vi "WFS Error Message.vi"(8 "error in (no error)":errorcluster {"code" format="%.0x"}, 10 "Error Code":i32 format="%.0g", 11 "instrument handle":refnum<visa-resource-name>) -> (0 "error out":errorcluster {"code" format="%.0x"}, 2 "Error Message":string, 3 "instrument handle out":refnum<visa-resource-name>)   [LabVIEW 2020]
doc: "This VI translates the error return value from a VXIplug&play instrument driver VI to a user-readable string."
uses:
  WFS_32.dll
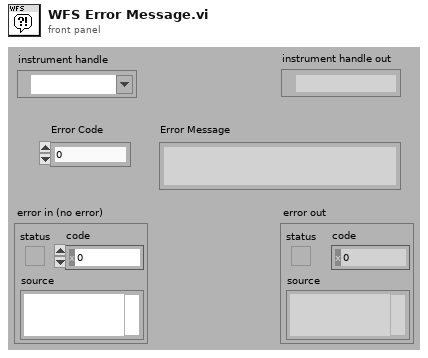
[diagram p1: front panel]
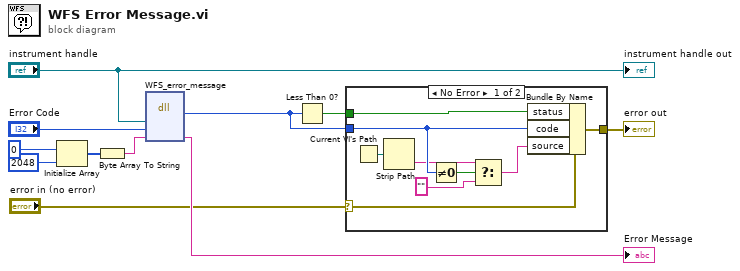
[diagram p0: block diagram]
diagram:
  n1 = Initialize Array(u8 0, 2048 ("size of error message")) -> (w9:u8[])
  n2 = Byte Array To String(unsigned byte array=w9) -> (string=w7:string)
  n3 = dll-call lib="WFS_*.*" fn="WFS_error_message"("instrument handle"="instrument handle", "error code"="Error Code", "error message"=w7) -> ("Status"=w2:i32, "error message"=→"Error Message":string)  [unwired: 5 in, 2 out]
  n4 = Less Than 0?(x=w2) -> (x < 0?=w3:bool)
  n5 = case shown="No Error" "error in (no error)" {
    selector: "error in (no error)" -> [w15 w21]
    tunnel: [w17 w21] -> w1
    tunnel: w3 -> [w18 _]
    tunnel: w2 -> [w14 _]
    frame No Error {
      n6 = Current VI's Path() -> (path=w13:path)
      n7 = Strip Path(path=w13) -> (name=w12:string)  [unwired: 1 out]
      n8 = Not Equal To 0?(x=w14) -> (x != 0?=w16:bool)
      n9 = Select(t=w12, s=w16, f="") -> (s? t:f=w19:string)
      n10 = Bundle By Name(cluster=w15, "status"=w18, "code"=w14, "source"=w19) -> (w17:errorcluster)
    }
    frame Error {
    }
  }
  "error out" <- w1
  "instrument handle out" <- "instrument handle"
